vi "Example.vi"() -> ()   [LabVIEW 2019, in "MicronCLI.lvclass"]
uses:
  MicronCLI.lvclass
  MicronCLI.lvclass/MicronCLI.ctl
  Typedefs/ServiceDetails.ctl
panel:
  out "Free Port Out":i64
  in  "Preferred Port":i64
  out "Version":string
  in  "ConnectionString":string="localhost:50051"
  in  "SkipIfNotPresent?":bool=TRUE
  in  "MicronCLI":path=path "micronCLI.exe"
  out "ConnectionStringBeforeRegister":string
  out "ConnectionStringAfterUnregister":string
  out "ConnectionStringAfterRegister":string
  in  "Service":T1={"Network"="mynetwork", "ServiceID"="myapp1"}
  out "error out":errorcluster
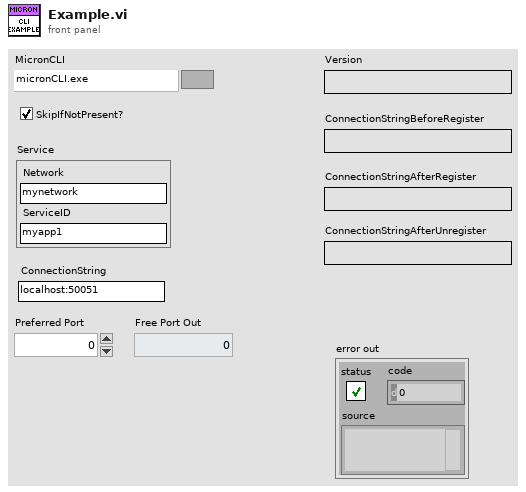
[diagram p1: front panel]
types:
  T1 = typedef "MicronCLI.lvclass/ServiceDetails.ctl" = cluster{"Network":string, "ServiceID":string}
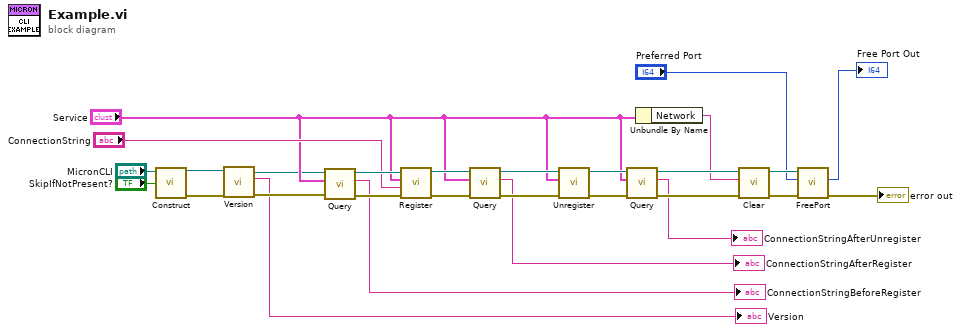
[diagram p0: block diagram]
diagram:
  n1 = call "Construct.vi"("SkipIfNotPresent?"="SkipIfNotPresent?", "MicronCLI"="MicronCLI") -> ("error out"=w10:errorcluster, "MicronCLI out"=w7:refnum<class "MicronCLI.lvclass">)  [unwired: 7 in, 1 out]
  n2 = call-dynamic "Version.vi"("error in (no error)"=w10, "MicronCLI in"=w7) -> ("error out"=w9:errorcluster, "Version"=→"Version":string, "MicronCLI out"=w8:refnum<class "MicronCLI.lvclass">)  [unwired: 7 in]
  n3 = call-dynamic "Query.vi"("error in (no error)"=w9, "Service"="Service", "MicronCLI in"=w8) -> ("error out"=w17:errorcluster, "ConnectionString"=→"ConnectionStringBeforeRegister":string, "MicronCLI out"=w18:refnum<class "MicronCLI.lvclass">)  [unwired: 6 in]
  n4 = call-dynamic "Register.vi"("error in (no error)"=w17, "ConnectionString"="ConnectionString", "Service"="Service", "MicronCLI in"=w18) -> ("error out"=w28:errorcluster, "MicronCLI out"=w27:refnum<class "MicronCLI.lvclass">)  [unwired: 6 in]
  n5 = call-dynamic "Query.vi"("error in (no error)"=w28, "Service"="Service", "MicronCLI in"=w27) -> ("error out"=w26:errorcluster, "ConnectionString"=→"ConnectionStringAfterRegister":string, "MicronCLI out"=w25:refnum<class "MicronCLI.lvclass">)  [unwired: 6 in]
  n6 = call-dynamic "Unregister.vi"("error in (no error)"=w26, "Service"="Service", "MicronCLI in"=w25) -> ("error out"=w24:errorcluster, "MicronCLI out"=w23:refnum<class "MicronCLI.lvclass">)  [unwired: 7 in]
  n7 = call-dynamic "Query.vi"("error in (no error)"=w24, "Service"="Service", "MicronCLI in"=w23) -> ("error out"=w22:errorcluster, "ConnectionString"=→"ConnectionStringAfterUnregister":string, "MicronCLI out"=w21:refnum<class "MicronCLI.lvclass">)  [unwired: 6 in]
  n8 = Unbundle By Name("Service") -> ("Network"=w11:string)
  n9 = call-dynamic "Clear.vi"("error in (no error)"=w22, "Network"=w11, "MicronCLI in"=w21) -> ("error out"=w5:errorcluster, "MicronCLI out"=w3:refnum<class "MicronCLI.lvclass">)  [unwired: 7 in]
  n10 = call-dynamic "FreePort.vi"("error in (no error)"=w5, "Port In"="Preferred Port", "MicronCLI in"=w3) -> ("error out"=→"error out":errorcluster, "Port Out"=→"Free Port Out":i64)  [unwired: 6 in, 1 out]
